vi "Show Ring.vi"(0 "Listbox":refnum<vi>, 1 "Ring":refnum<vi>, 5 "item":T2, 9 "cell":T1, 11 "error in (no error)":errorcluster) -> (15 "error out":errorcluster)   [LabVIEW 2015]
uses:
  RowData.ctl
  DataType.ctl
  <vilib>/Utility/miscctls.llb/LVRowAndColumnTypeDef.ctl
  KPropertyTable.xctl
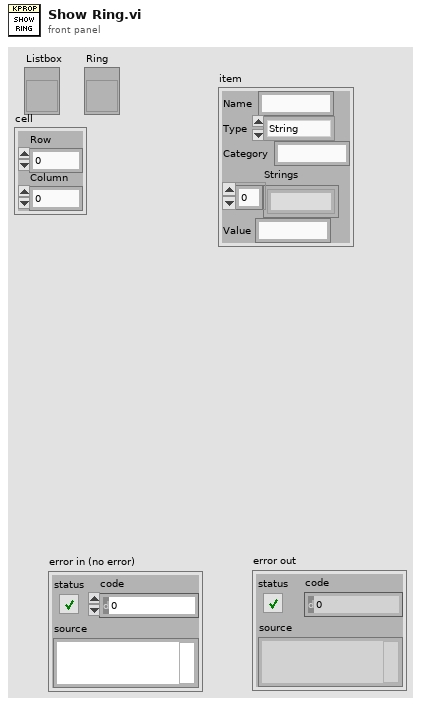
[diagram p1: front panel]
types:
  T1 = typedef "LVRowAndColumnTypeDef.ctl" = cluster{"Row":i32, "Column":i32}
  T2 = typedef "KPropertyTable.xctl/RowData.ctl" = cluster{"Name":string, "Type":T3, "Category":string, "Strings":string[], "Value":string}
  T3 = typedef "KPropertyTable.xctl/DataType.ctl" = enum16{"String", "Enum", "Int", "Double", "Boolean", "Ring", "Formula"}
  T4 = typedef "LVPositionTypeDef.ctl" = cluster{"Left":i32, "Top":i32}
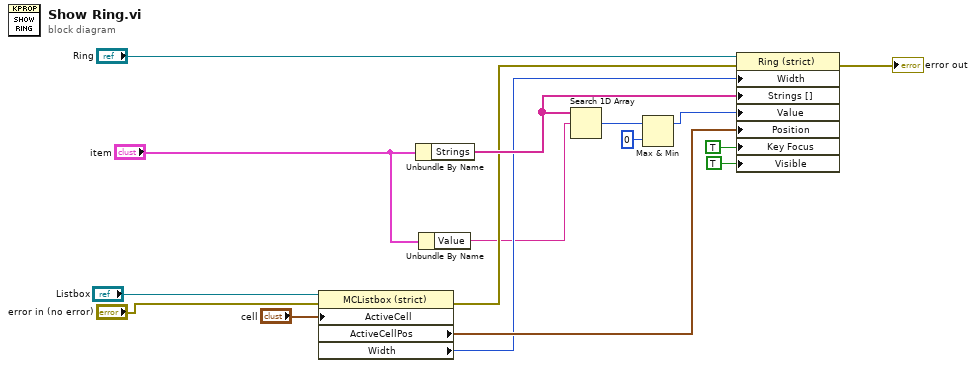
[diagram p0: block diagram]
diagram:
  n1 = property class="MCListbox (strict)"(reference="Listbox", error in="error in (no error)", "ActiveCell"="cell") -> (error out=w11:errorcluster, "ActiveCellPos"=w13:T4, "Width"=w9:u32)  [unwired: 1 out]
  n2 = Unbundle By Name("item") -> ("Strings"=w12:string[])
  n3 = Unbundle By Name("item") -> ("Value"=w8:string)
  n4 = Search 1D Array(1D array=w12, element=w8) -> (index of element=w2:i32)  [unwired: 1 in]
  n5 = Max & Min(x=w2, y=0) -> (max(x,y)=w3:i32)  [unwired: 1 out]
  n6 = property on="Property Node" class="Ring (strict)"(reference="Ring", error in=w11, "Width"=w9, "Strings []"=w12, "Value"=w3, "Position"=w13, "Key Focus"=TRUE, "Visible"=TRUE) -> (error out=→"error out":errorcluster)  [unwired: 1 out]
